vi "FL_DEC_split.vi"(0 "InputArray":sgl[](array[numeric])) -> (4 "X1":sgl, 5 "Y1":sgl, 6 "X2":sgl, 7 "Y2":sgl)   [LabVIEW 2018, in "Tracker.lvlib"]
uses:
  Tracker.lvlib
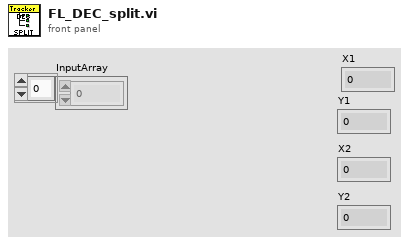
[diagram p1: front panel]
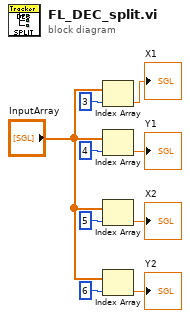
[diagram p0: block diagram]
diagram:
  n1 = Index Array(array="InputArray", index=3 ("disabled index (col)")) -> (element=→"X1":sgl)
  n2 = Index Array(array="InputArray", index=4 ("disabled index (col)")) -> (element=→"Y1":sgl)
  n3 = Index Array(array="InputArray", index=5 ("disabled index (col)")) -> (element=→"X2":sgl)
  n4 = Index Array(array="InputArray", index=6 ("disabled index (col)")) -> (element=→"Y2":sgl)
